vi "array -- fold to mon increasing.vi"(11 "Array":dbl[](array[numeric])) -> (3 "Array out":dbl[](array[numeric]))   [LabVIEW 2012]
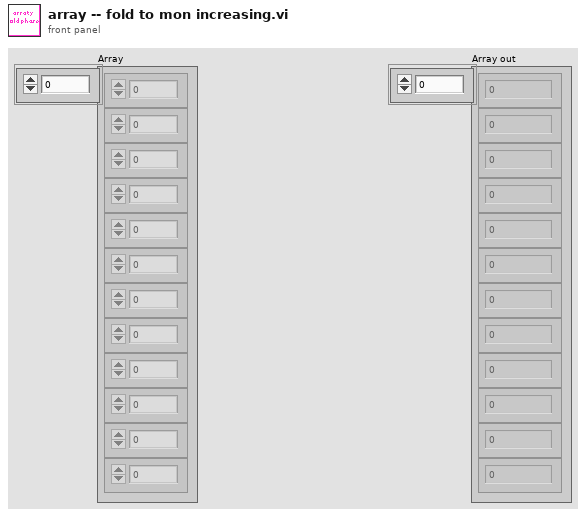
[diagram p1: front panel]
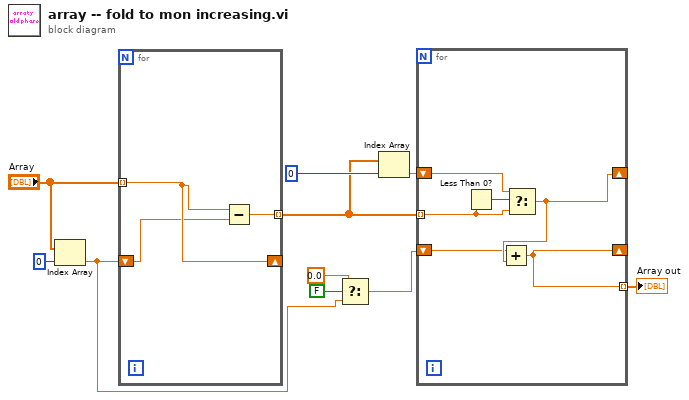
[diagram p0: block diagram]
diagram:
  n1 = Index Array(array="Array", index=0) -> (element=w2:dbl)
  n2 = for {
    tunnel: "Array" -> [w13] mode=indexing
    shift-right: [w13] -> _
    shift-left: w2 -> [w12]
    tunnel: [w11] -> w7 mode=indexing
    n3 = Subtract(x=w13, y=w12) -> (x-y=w11:dbl)
  }
  n4 = Select(t=0.0, s=FALSE, f=w2) -> (s? t:f=w1:dbl)
  n5 = Index Array(array=w7, index=0) -> (element=w6:dbl)
  n6 = for {
    tunnel: w7 -> [w14] mode=indexing
    shift-right: [w18] -> _
    shift-left: w6 -> [w15]
    shift-right: [w16] -> _
    shift-left: w1 -> [w17]
    tunnel: [w16] -> w5 mode=indexing
    n7 = Less Than 0?(x=w14) -> (x < 0?=w19:bool)
    n8 = Select(t=w15, s=w19, f=w14) -> (s? t:f=w18:dbl)
    n9 = Add(x=w17, y=w18) -> (x+y=w16:dbl)
  }
  "Array out" <- w5
